vi "Trial 3 A4.vi"() -> ()   [LabVIEW 2022 SP3]
uses:
  Documents/Control 1 Trial 3.ctl
panel:
  in  "Washing Mode Menu":T1(ring)
  in  "Start":bool
  out "Washing Stage":string
  out "Washing Mode":string
  out "Time remaining":dbl
  in  "On/Off":bool
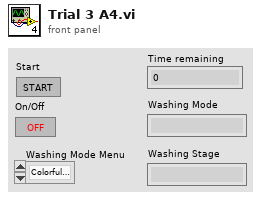
[diagram p1: front panel]
types:
  T1 = enum16{"Colorful Mode", "Intensive Mode", "Quick Wash", ""}
  T2 = typedef "Control 1 Trial 3.ctl" = enum16{"Off", "On", "Start Washing", "Pre-rinse", "Main Washing", "Final Spin", "Done Washing"}
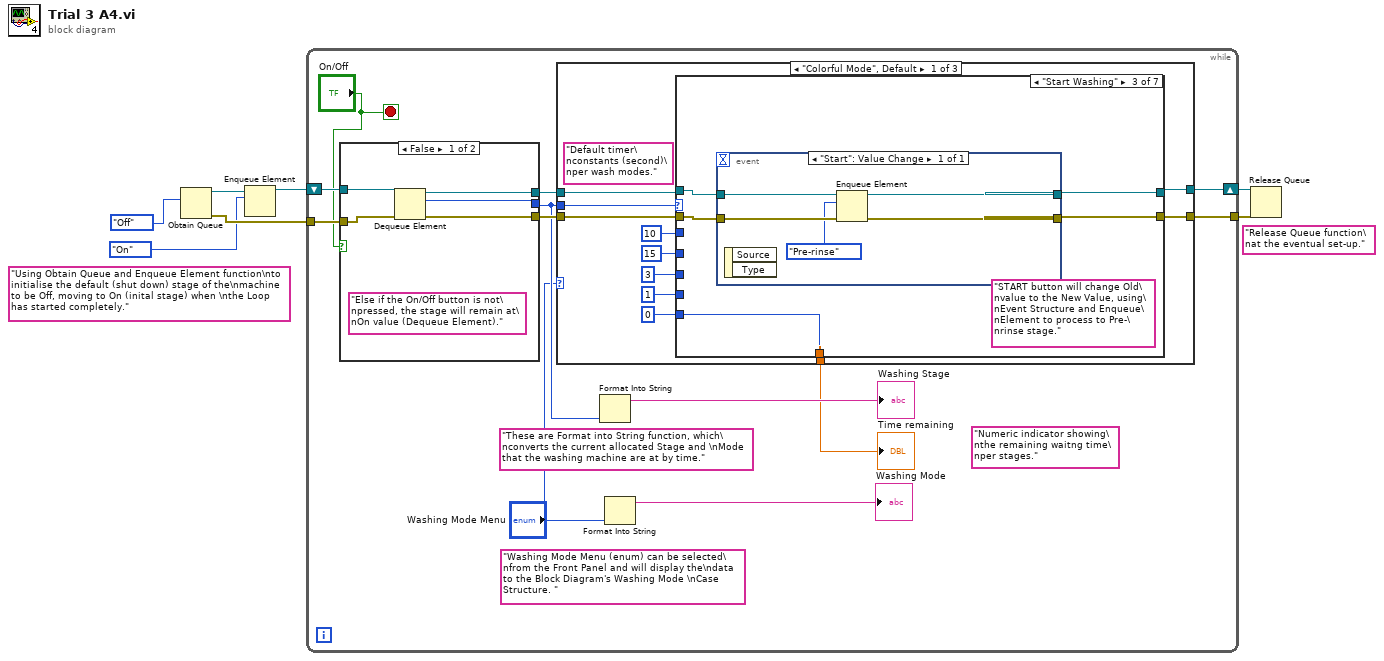
[diagram p0: block diagram]
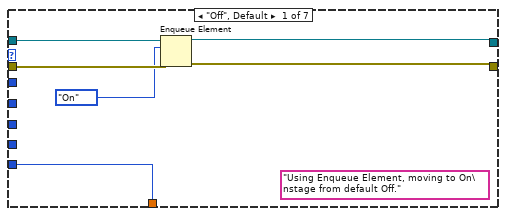
[diagram p2: hidden frame]
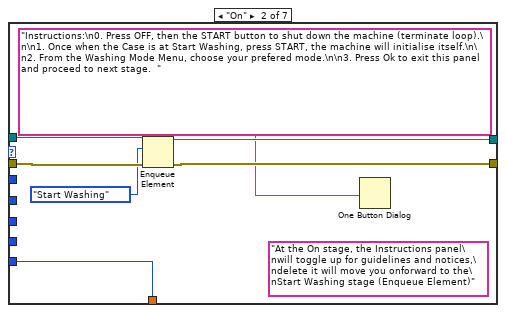
[diagram p3: hidden frame]
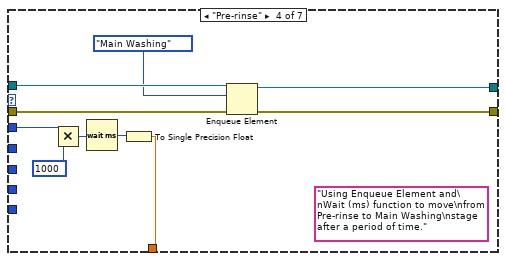
[diagram p4: hidden frame]
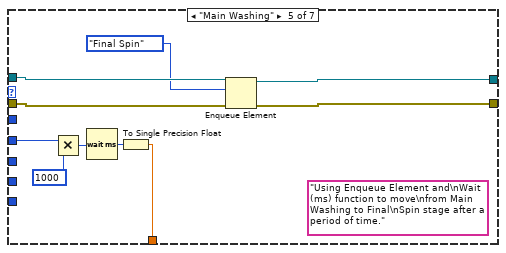
[diagram p5: hidden frame]
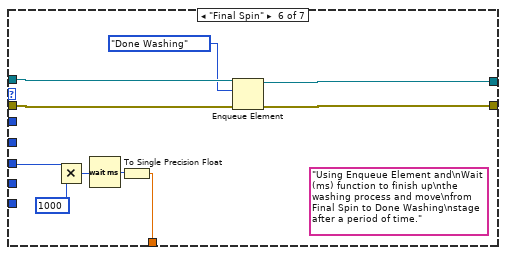
[diagram p6: hidden frame]
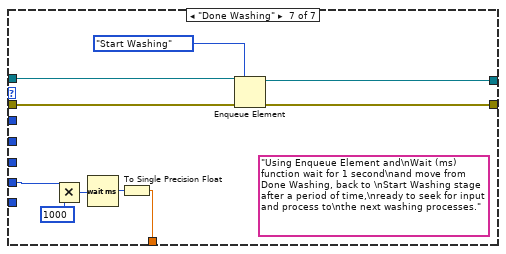
[diagram p7: hidden frame]
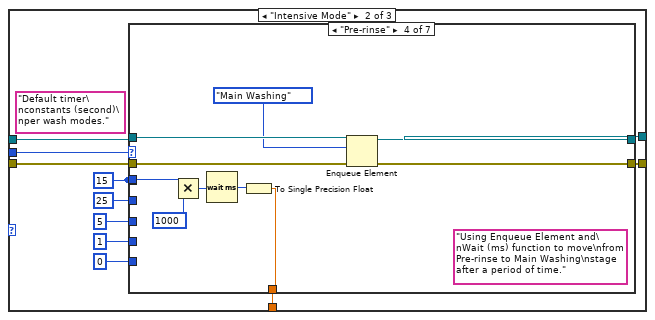
[diagram p8: hidden frame]
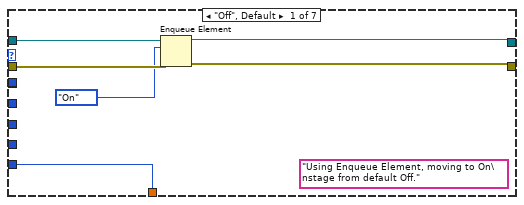
[diagram p9: hidden frame]
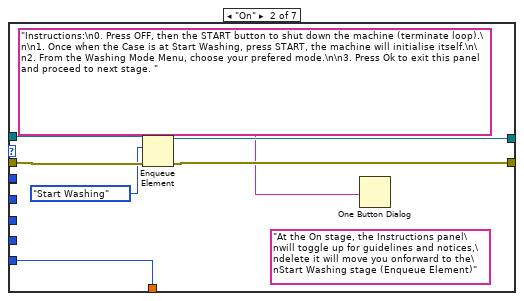
[diagram p10: hidden frame]
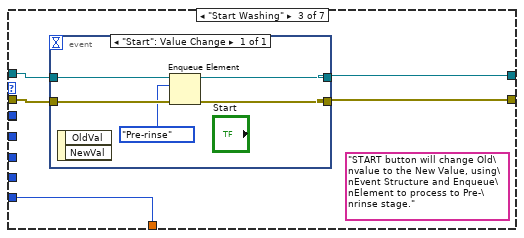
[diagram p11: hidden frame]
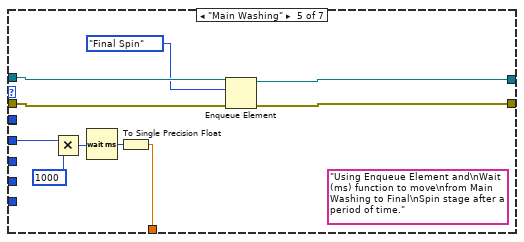
[diagram p12: hidden frame]
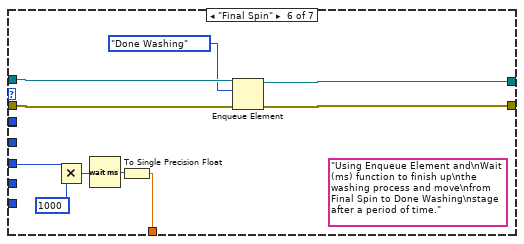
[diagram p13: hidden frame]
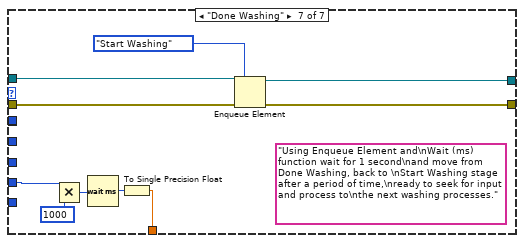
[diagram p14: hidden frame]
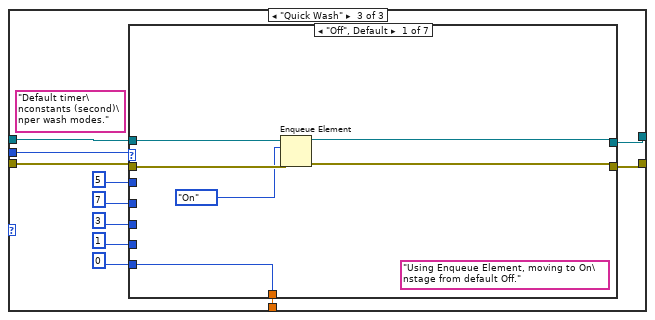
[diagram p15: hidden frame]
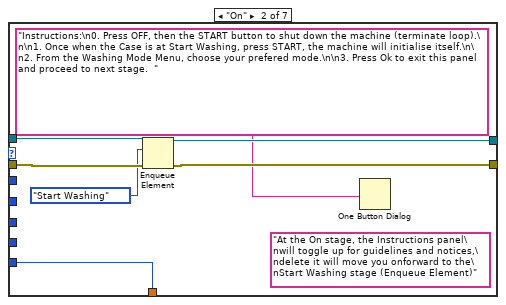
[diagram p16: hidden frame]
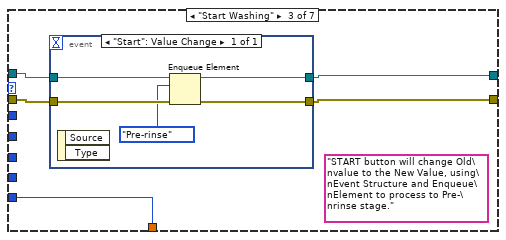
[diagram p17: hidden frame]
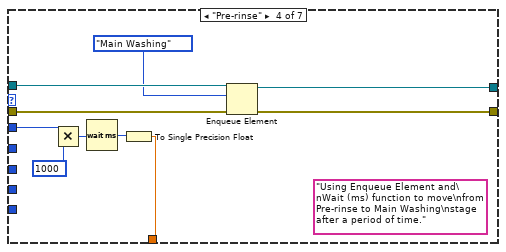
[diagram p18: hidden frame]
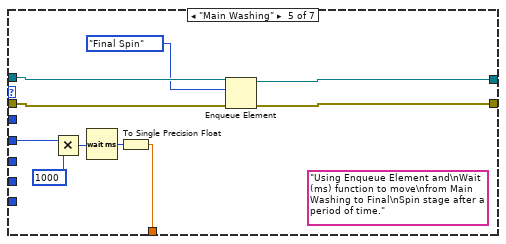
[diagram p19: hidden frame]
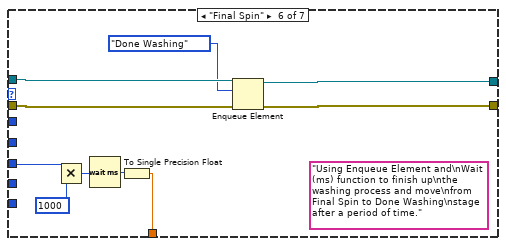
[diagram p20: hidden frame]
diagram:
  (unwired) "Release Queue function\nat the eventual set-up."
  (unwired) "Using Obtain Queue and Enqueue Element function\nto initialise the default (shut down) stage of the\nmachine to be Off, moving to On (inital stage) when \nthe Loop has started completely."
  n1 = Obtain Queue(element data type=Control_1_Trial_3."Off") -> (queue out=w7:refnum<queue>, error out=w5:errorcluster)  [unwired: 4 in, 1 out]
  n2 = Enqueue Element(queue=w7, element=Control_1_Trial_3."On") -> (queue out=w6:refnum<queue>)  [unwired: 2 in, 2 out]
  n3 = while {
    shift-right: [w15] -> w3
    shift-left: w6 -> [w18]
    tunnel: w5 -> [w19]
    tunnel: [w13] -> w4
    stop <- "On/Off" stop-if-true
    (unwired) "Numeric indicator showing\nthe remaining waitng time\nper stages."
    (unwired) "Washing Mode Menu (enum) can be selected\nfrom the Front Panel and will display the\ndata to the Block Diagram's Washing Mode \nCase Structure. "
    (unwired) "These are Format into String function, which\nconverts the current allocated Stage and \nMode that the washing machine are at by time."
    n4 = case shown="False" "On/Off" {
      tunnel: w19 -> [w244 w250]
      tunnel: w18 -> [w246 w251]
      tunnel: [w245 w249] -> w16
      tunnel: [w243 w248] -> w14
      tunnel: [w242 Control_1_Trial_3."Off"] -> w11
      frame False {
        (unwired) "Else if the On/Off button is not\npressed, the stage will remain at\nOn value (Dequeue Element)."
        n5 = Dequeue Element(queue=w246, error in (no error)=w244) -> (queue out=w245:refnum<queue>, element=w242:T2, error out=w243:errorcluster)  [unwired: 1 in, 1 out]
      }
      frame True {
        (unwired) "If the On/Off button is pressed,\nthe Stage immidiately go to Off,\nwhich also means the machine\nhas been shut down and restarted\nonce when the loop is back (Flush\nQueue element toggled)."
        n6 = Flush Queue(queue=w251, error in (no error)=w250) -> (queue out=w249:refnum<queue>, error out=w248:errorcluster)  [unwired: 1 out]
      }
    }
    n7 = case shown="\"Colorful Mode\", Default" "Washing Mode Menu" {
      tunnel: w16 -> [w30 w104 w177]
      tunnel: [w27 w103 w174] -> w15
      tunnel: w14 -> [w29 w102 w176]
      tunnel: [w26 w101 w173] -> w13
      tunnel: [w20 w100 w178] -> w12
      tunnel: w11 -> [w28 w99 w175]
      frame "Colorful Mode", Default {
        (unwired) "Default timer\nconstants (second)\nper wash modes."
        n8 = case shown="\"Start Washing\"" w28 {
          tunnel: w30 -> [w36 w43 w48 w63 w73 w83 w91]
          tunnel: [w33 w42 w47 w61 w71 w81 w93] -> w27
          tunnel: w29 -> [w35 w41 w46 w62 w72 w82 w90]
          tunnel: [w34 w40 w45 w60 w70 w80 w92] -> w26
          tunnel: [w31 w37 w44 w55 w64 w74 w84] -> w20
          tunnel: 15 -> [_ _ _ _ w66 _ _]
          tunnel: 3 -> [_ _ _ _ _ w76 _]
          tunnel: 1 -> [_ _ _ _ _ _ w86]
          tunnel: 0 -> [w31 w37 w44 _ _ _ _]
          tunnel: 10 -> [_ _ _ w58 _ _ _]
          frame "Off", Default {
            (unwired) "Using Enqueue Element, moving to On\nstage from default Off."
            n9 = Enqueue Element(queue=w36, element=Control_1_Trial_3."On", error in (no error)=w35) -> (queue out=w33:refnum<queue>, error out=w34:errorcluster)  [unwired: 1 in, 1 out]
          }
          frame "On" {
            (unwired) "At the On stage, the Instructions panel\nwill toggle up for guidelines and notices,\ndelete it will move you onforward to the\nStart Washing stage (Enqueue Element)"
            n10 = Enqueue Element(queue=w43, element=Control_1_Trial_3."Start Washing", error in (no error)=w41) -> (queue out=w42:refnum<queue>, error out=w40:errorcluster)  [unwired: 1 in, 1 out]
            n11 = One Button Dialog(message="Instructions:\n0. Press OFF, then the START button to shut down the machine (terminate loop).\n\n1. Once when the Case is at Start Washing, press START, the machine will initialise itself.\n\n2. From the Washing Mode Menu, choose your prefered mode.\n\n3. Press Ok to exit this panel and proceed to next stage.  ") -> ()  [unwired: 1 in, 1 out]
          }
          frame "Start Washing" {
            (unwired) "START button will change Old\nvalue to the New Value, using\nEvent Structure and Enqueue\nElement to process to Pre-\nrinse stage."
            n12 = event shown="[0] \"Start\": Value Change" {
              selector: _ -> [_]
              dyn-events: _ -> [_]
              timeout: _ -> [_]
              tunnel: w48 -> [w53]
              tunnel: [w52] -> w47
              tunnel: w46 -> [w51]
              tunnel: [w50] -> w45
              event "Start": Value Change {
                n13 = event-data() -> ()  [unwired: 1 in, 2 out]
                n14 = Enqueue Element(queue=w53, element=Control_1_Trial_3."Pre-rinse", error in (no error)=w51) -> (queue out=w52:refnum<queue>, error out=w50:errorcluster)  [unwired: 1 in, 1 out]
              }
            }
          }
          frame "Pre-rinse" {
            (unwired) "Using Enqueue Element and\nWait (ms) function to move\nfrom Pre-rinse to Main Washing\nstage after a period of time."
            n15 = Multiply(x=w58, y=1000) -> (x*y=w56:i32)
            n16 = Wait (ms)(milliseconds to wait=w56) -> (millisecond timer value=w54:u32)
            n17 = To Single Precision Float(number=w54) -> (single precision float=w55:sgl)
            n18 = Enqueue Element(queue=w63, element=Control_1_Trial_3."Main Washing", error in (no error)=w62) -> (queue out=w61:refnum<queue>, error out=w60:errorcluster)  [unwired: 1 in, 1 out]
          }
          frame "Main Washing" {
            (unwired) "Using Enqueue Element and\nWait (ms) function to move\nfrom Main Washing to Final\nSpin stage after a period of time."
            n19 = Multiply(x=w66, y=1000) -> (x*y=w67:i32)
            n20 = Wait (ms)(milliseconds to wait=w67) -> (millisecond timer value=w65:u32)
            n21 = To Single Precision Float(number=w65) -> (single precision float=w64:sgl)
            n22 = Enqueue Element(queue=w73, element=Control_1_Trial_3."Final Spin", error in (no error)=w72) -> (queue out=w71:refnum<queue>, error out=w70:errorcluster)  [unwired: 1 in, 1 out]
          }
          frame "Final Spin" {
            (unwired) "Using Enqueue Element and\nWait (ms) function to finish up\nthe washing process and move\nfrom Final Spin to Done Washing\nstage after a period of time."
            n23 = Multiply(x=w76, y=1000) -> (x*y=w77:i32)
            n24 = Wait (ms)(milliseconds to wait=w77) -> (millisecond timer value=w75:u32)
            n25 = To Single Precision Float(number=w75) -> (single precision float=w74:sgl)
            n26 = Enqueue Element(queue=w83, element=Control_1_Trial_3."Done Washing", error in (no error)=w82) -> (queue out=w81:refnum<queue>, error out=w80:errorcluster)  [unwired: 1 in, 1 out]
          }
          frame "Done Washing" {
            (unwired) "Using Enqueue Element and\nWait (ms) function wait for 1 second\nand move from Done Washing, back to \nStart Washing stage after a period of time,\nready to seek for input and process to\nthe next washing processes."
            n27 = Multiply(x=w86, y=1000) -> (x*y=w87:i32)
            n28 = Wait (ms)(milliseconds to wait=w87) -> (millisecond timer value=w85:u32)
            n29 = To Single Precision Float(number=w85) -> (single precision float=w84:sgl)
            n30 = Enqueue Element(queue=w91, element=Control_1_Trial_3."Start Washing", error in (no error)=w90) -> (queue out=w93:refnum<queue>, error out=w92:errorcluster)  [unwired: 1 in, 1 out]
          }
        }
      }
      frame "Intensive Mode" {
        (unwired) "Default timer\nconstants (second)\nper wash modes."
        w94 = 15
        n31 = case shown="\"Pre-rinse\"" w99 {
          tunnel: w104 -> [w110 w117 w122 w137 w147 w157 w165]
          tunnel: [w107 w116 w121 w135 w145 w155 w167] -> w103
          tunnel: w102 -> [w109 w115 w120 w136 w146 w156 w164]
          tunnel: [w108 w114 w119 w134 w144 w154 w166] -> w101
          tunnel: [w105 w111 w118 w129 w138 w148 w158] -> w100
          tunnel: w94 -> [_ _ _ _ _ _ _]
          tunnel: 25 -> [_ _ _ _ w140 _ _]
          tunnel: 5 -> [_ _ _ _ _ w150 _]
          tunnel: 1 -> [_ _ _ _ _ _ w160]
          tunnel: 0 -> [w105 w111 w118 _ _ _ _]
          tunnel: w94 -> [_ _ _ w132 _ _ _]
          frame "Off", Default {
            (unwired) "Using Enqueue Element, moving to On\nstage from default Off."
            n32 = Enqueue Element(queue=w110, element=Control_1_Trial_3."On", error in (no error)=w109) -> (queue out=w107:refnum<queue>, error out=w108:errorcluster)  [unwired: 1 in, 1 out]
          }
          frame "On" {
            (unwired) "At the On stage, the Instructions panel\nwill toggle up for guidelines and notices,\ndelete it will move you onforward to the\nStart Washing stage (Enqueue Element)"
            n33 = Enqueue Element(queue=w117, element=Control_1_Trial_3."Start Washing", error in (no error)=w115) -> (queue out=w116:refnum<queue>, error out=w114:errorcluster)  [unwired: 1 in, 1 out]
            n34 = One Button Dialog(message="Instructions:\n0. Press OFF, then the START button to shut down the machine (terminate loop).\n\n1. Once when the Case is at Start Washing, press START, the machine will initialise itself.\n\n2. From the Washing Mode Menu, choose your prefered mode.\n\n3. Press Ok to exit this panel and proceed to next stage. ") -> ()  [unwired: 1 in, 1 out]
          }
          frame "Start Washing" {
            (unwired) "START button will change Old\nvalue to the New Value, using\nEvent Structure and Enqueue\nElement to process to Pre-\nrinse stage."
            n35 = event shown="[0] \"Start\": Value Change" {
              selector: _ -> [_]
              dyn-events: _ -> [_]
              timeout: _ -> [_]
              tunnel: w122 -> [w127]
              tunnel: [w126] -> w121
              tunnel: w120 -> [w125]
              tunnel: [w124] -> w119
              event "Start": Value Change {
                n36 = event-data() -> ()  [unwired: 1 in, 2 out]
                n37 = Enqueue Element(queue=w127, element=Control_1_Trial_3."Pre-rinse", error in (no error)=w125) -> (queue out=w126:refnum<queue>, error out=w124:errorcluster)  [unwired: 1 in, 1 out]
              }
            }
          }
          frame "Pre-rinse" {
            (unwired) "Using Enqueue Element and\nWait (ms) function to move\nfrom Pre-rinse to Main Washing\nstage after a period of time."
            n38 = Multiply(x=w132, y=1000) -> (x*y=w130:i32)
            n39 = Wait (ms)(milliseconds to wait=w130) -> (millisecond timer value=w128:u32)
            n40 = To Single Precision Float(number=w128) -> (single precision float=w129:sgl)
            n41 = Enqueue Element(queue=w137, element=Control_1_Trial_3."Main Washing", error in (no error)=w136) -> (queue out=w135:refnum<queue>, error out=w134:errorcluster)  [unwired: 1 in, 1 out]
          }
          frame "Main Washing" {
            (unwired) "Using Enqueue Element and\nWait (ms) function to move\nfrom Main Washing to Final\nSpin stage after a period of time."
            n42 = Multiply(x=w140, y=1000) -> (x*y=w141:i32)
            n43 = Wait (ms)(milliseconds to wait=w141) -> (millisecond timer value=w139:u32)
            n44 = To Single Precision Float(number=w139) -> (single precision float=w138:sgl)
            n45 = Enqueue Element(queue=w147, element=Control_1_Trial_3."Final Spin", error in (no error)=w146) -> (queue out=w145:refnum<queue>, error out=w144:errorcluster)  [unwired: 1 in, 1 out]
          }
          frame "Final Spin" {
            (unwired) "Using Enqueue Element and\nWait (ms) function to finish up\nthe washing process and move\nfrom Final Spin to Done Washing\nstage after a period of time."
            n46 = Multiply(x=w150, y=1000) -> (x*y=w151:i32)
            n47 = Wait (ms)(milliseconds to wait=w151) -> (millisecond timer value=w149:u32)
            n48 = To Single Precision Float(number=w149) -> (single precision float=w148:sgl)
            n49 = Enqueue Element(queue=w157, element=Control_1_Trial_3."Done Washing", error in (no error)=w156) -> (queue out=w155:refnum<queue>, error out=w154:errorcluster)  [unwired: 1 in, 1 out]
          }
          frame "Done Washing" {
            (unwired) "Using Enqueue Element and\nWait (ms) function wait for 1 second\nand move from Done Washing, back to \nStart Washing stage after a period of time,\nready to seek for input and process to\nthe next washing processes."
            n50 = Multiply(x=w160, y=1000) -> (x*y=w161:i32)
            n51 = Wait (ms)(milliseconds to wait=w161) -> (millisecond timer value=w159:u32)
            n52 = To Single Precision Float(number=w159) -> (single precision float=w158:sgl)
            n53 = Enqueue Element(queue=w165, element=Control_1_Trial_3."Start Washing", error in (no error)=w164) -> (queue out=w167:refnum<queue>, error out=w166:errorcluster)  [unwired: 1 in, 1 out]
          }
        }
      }
      frame "Quick Wash" {
        (unwired) "Default timer\nconstants (second)\nper wash modes."
        n54 = case shown="\"Off\", Default" w175 {
          tunnel: w177 -> [w184 w191 w196 w211 w221 w231 w239]
          tunnel: [w181 w190 w195 w209 w219 w229 w241] -> w174
          tunnel: w176 -> [w183 w189 w194 w210 w220 w230 w238]
          tunnel: [w182 w188 w193 w208 w218 w228 w240] -> w173
          tunnel: [w179 w185 w192 w203 w212 w222 w232] -> w178
          tunnel: 7 -> [_ _ _ _ w214 _ _]
          tunnel: 3 -> [_ _ _ _ _ w224 _]
          tunnel: 1 -> [_ _ _ _ _ _ w234]
          tunnel: 0 -> [w179 w185 w192 _ _ _ _]
          tunnel: 5 -> [_ _ _ w206 _ _ _]
          frame "Off", Default {
            (unwired) "Using Enqueue Element, moving to On\nstage from default Off."
            n55 = Enqueue Element(queue=w184, element=Control_1_Trial_3."On", error in (no error)=w183) -> (queue out=w181:refnum<queue>, error out=w182:errorcluster)  [unwired: 1 in, 1 out]
          }
          frame "On" {
            (unwired) "At the On stage, the Instructions panel\nwill toggle up for guidelines and notices,\ndelete it will move you onforward to the\nStart Washing stage (Enqueue Element)"
            n56 = Enqueue Element(queue=w191, element=Control_1_Trial_3."Start Washing", error in (no error)=w189) -> (queue out=w190:refnum<queue>, error out=w188:errorcluster)  [unwired: 1 in, 1 out]
            n57 = One Button Dialog(message="Instructions:\n0. Press OFF, then the START button to shut down the machine (terminate loop).\n\n1. Once when the Case is at Start Washing, press START, the machine will initialise itself.\n\n2. From the Washing Mode Menu, choose your prefered mode.\n\n3. Press Ok to exit this panel and proceed to next stage.  ") -> ()  [unwired: 1 in, 1 out]
          }
          frame "Start Washing" {
            (unwired) "START button will change Old\nvalue to the New Value, using\nEvent Structure and Enqueue\nElement to process to Pre-\nrinse stage."
            n58 = event shown="[0] \"Start\": Value Change" {
              selector: _ -> [_]
              dyn-events: _ -> [_]
              timeout: _ -> [_]
              tunnel: w196 -> [w201]
              tunnel: [w200] -> w195
              tunnel: w194 -> [w199]
              tunnel: [w198] -> w193
              event "Start": Value Change {
                n59 = event-data() -> ()  [unwired: 1 in, 2 out]
                n60 = Enqueue Element(queue=w201, element=Control_1_Trial_3."Pre-rinse", error in (no error)=w199) -> (queue out=w200:refnum<queue>, error out=w198:errorcluster)  [unwired: 1 in, 1 out]
              }
            }
          }
          frame "Pre-rinse" {
            (unwired) "Using Enqueue Element and\nWait (ms) function to move\nfrom Pre-rinse to Main Washing\nstage after a period of time."
            n61 = Multiply(x=w206, y=1000) -> (x*y=w204:i32)
            n62 = Wait (ms)(milliseconds to wait=w204) -> (millisecond timer value=w202:u32)
            n63 = To Single Precision Float(number=w202) -> (single precision float=w203:sgl)
            n64 = Enqueue Element(queue=w211, element=Control_1_Trial_3."Main Washing", error in (no error)=w210) -> (queue out=w209:refnum<queue>, error out=w208:errorcluster)  [unwired: 1 in, 1 out]
          }
          frame "Main Washing" {
            (unwired) "Using Enqueue Element and\nWait (ms) function to move\nfrom Main Washing to Final\nSpin stage after a period of time."
            n65 = Multiply(x=w214, y=1000) -> (x*y=w215:i32)
            n66 = Wait (ms)(milliseconds to wait=w215) -> (millisecond timer value=w213:u32)
            n67 = To Single Precision Float(number=w213) -> (single precision float=w212:sgl)
            n68 = Enqueue Element(queue=w221, element=Control_1_Trial_3."Final Spin", error in (no error)=w220) -> (queue out=w219:refnum<queue>, error out=w218:errorcluster)  [unwired: 1 in, 1 out]
          }
          frame "Final Spin" {
            (unwired) "Using Enqueue Element and\nWait (ms) function to finish up\nthe washing process and move\nfrom Final Spin to Done Washing\nstage after a period of time."
            n69 = Multiply(x=w224, y=1000) -> (x*y=w225:i32)
            n70 = Wait (ms)(milliseconds to wait=w225) -> (millisecond timer value=w223:u32)
            n71 = To Single Precision Float(number=w223) -> (single precision float=w222:sgl)
            n72 = Enqueue Element(queue=w231, element=Control_1_Trial_3."Done Washing", error in (no error)=w230) -> (queue out=w229:refnum<queue>, error out=w228:errorcluster)  [unwired: 1 in, 1 out]
          }
          frame "Done Washing" {
            (unwired) "Using Enqueue Element and\nWait (ms) function wait for 1 second\nand move from Done Washing, back to \nStart Washing stage after a period of time,\nready to seek for input and process to\nthe next washing processes."
            n73 = Multiply(x=w234, y=1000) -> (x*y=w235:i32)
            n74 = Wait (ms)(milliseconds to wait=w235) -> (millisecond timer value=w233:u32)
            n75 = To Single Precision Float(number=w233) -> (single precision float=w232:sgl)
            n76 = Enqueue Element(queue=w239, element=Control_1_Trial_3."Start Washing", error in (no error)=w238) -> (queue out=w241:refnum<queue>, error out=w240:errorcluster)  [unwired: 1 in, 1 out]
          }
        }
      }
    }
    "Time remaining" <- w12
    n77 = Format Into String(w11) -> (resulting string=→"Washing Stage":string)  [unwired: 3 in, 1 out]
    n78 = Format Into String("Washing Mode Menu") -> (resulting string=→"Washing Mode":string)  [unwired: 3 in, 1 out]
  }
  n79 = Release Queue(queue=w3, error in (no error)=w4) -> ()  [unwired: 1 in, 3 out]
